vi "PM5000_ReadG6.vi"(6 "DEMO":bool=TRUE, 7 "ID_MEDICION":i32, 8 "error in (no error)":errorcluster, 10 "Equipo_Medicion":T1) -> (0 "error out":errorcluster, 2 "PM_out":T2={"Equipo_Medicion"={"ID_EQUIPO"=0, "IP_EQUIPO"="", "NOMBRE_EQUIPO"="", "ESTADO_EQUIPO"="", "DESCRIPCION"="", "ID_MEDICION"=0, "ESTADO_MEDICION"="", "TIEMPO_MEDICION"="12-02-2019 18:41"}, "VIF_cluster"={"VL_VL"={"V1_V2"=0.0, "V2_V3"=0.0, "V3_V1"=0.0, "Avg_VL_VL"=0.0}, "IL_IL"={"I1"=0.0, "I2"=0.0, "I3"=0.0, "Avg_Amps"=0.0}, "Frecuency"=0.0, "Avg_Frecuency"=0.0}, "Power_cluster"={"Real Power (kW)"={"L1_kW"=0.0, "L2_kW"=0.0, "L3_kW"=0.0, "Total_kW"=0.0}, "Reactive Power (kVAR)"={"L1_kVAR"=0.0, "L2_kVAR"=0.0, "L3_kVAR"=0.0, "Total_kVAR"=0.0}, "Aparent Power (kVA)"={"L1_kVA"=0.0, "L2_kVA"=0.0, "L3_kVA"=0.0, "Total_kVA"=0.0}, "Power Factor (%)"={"L1_PF"=0.0, "L2_PF"=0.0, "L3_PF"=0.0, "Total_PF"=0.0}}, "THD_cluster"={"V_THD"={"V1_V2_THD"=0.0, "V2_V3_THD"=0.0, "V3_V1_THD"=0.0, "Avg_V_V_THD"=0.0}, "I_THD"={"I1_THD"=0.0, "I2_THD"=0.0, "I3_THD"=0.0, "I4_THD"=0.0, "Avg_I_THD"=0.0}}, "Polar_cluster"={"V_polar"={"V1_ang"=0.0, "V1_mag"=0.0, "V2_ang"=0.0, "V2_mag"=0.0, "V3_ang"=0.0, "V3_mag"=0.0}, "I_polar"={"I1_ang"=0.0, "I1_mag"=0.0, "I2_ang"=0.0, "I2_mag"=0.0, "I3_ang"=0.0, "I3_mag"=0.0}}})   [LabVIEW 2018]
uses:
  Controls/Cluster_Data.ctl
  Controls/Equipos_Medicion_cluster.ctl
  Controls/VIF_cluster.ctl
  Controls/Power_cluster.ctl
  Controls/THD_cluster.ctl
  Controls/Polar_cluster.ctl
  Controls/Cluster_HMI_VIFP - 2.ctl
  <vilib>/RAFA Solutions/Harmony UI Controls Kit/Numeric/Horizontal Progress Bar.ctl
  <vilib>/RAFA Solutions/Harmony UI Controls Kit/Numeric/Numeric Indicator.ctl
  Global/globalGenerador6_HMI.vi
  <vilib>/RAFA Solutions/Harmony UI Controls Kit/Flat UI Design.lvlib
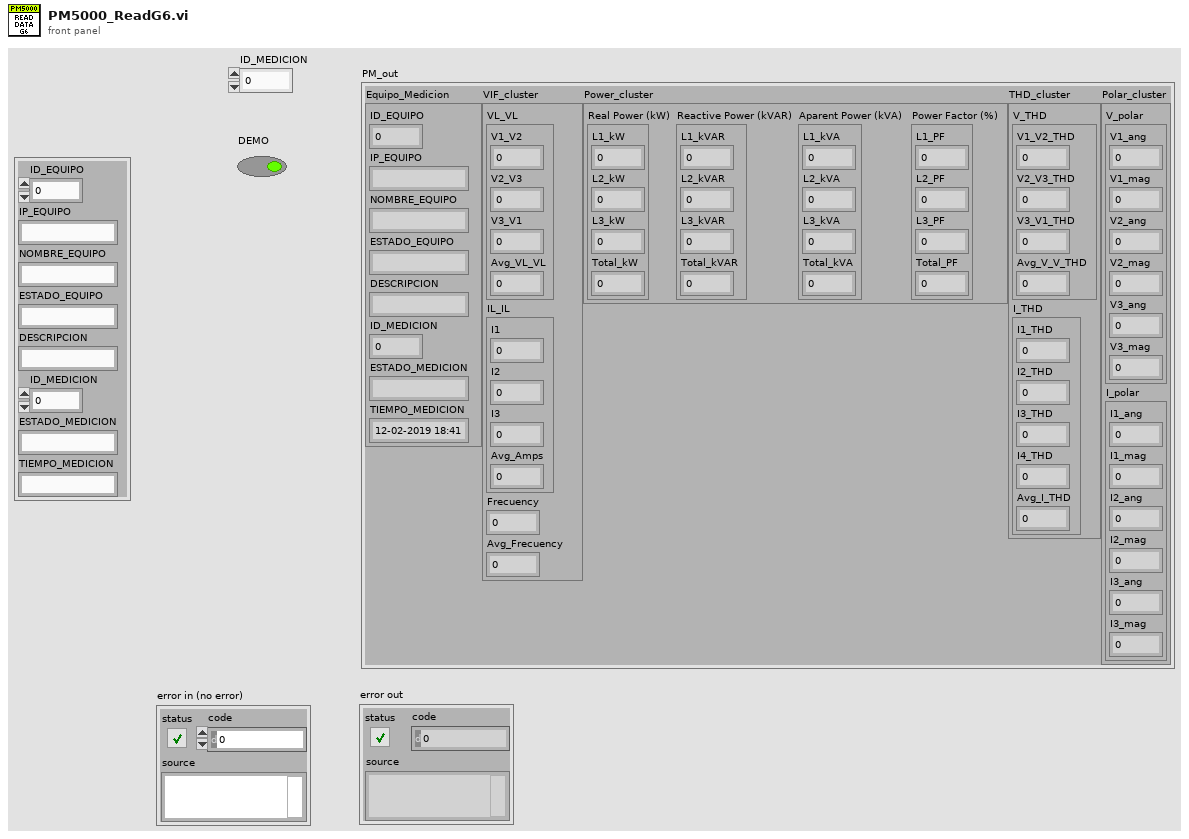
[diagram p1: front panel]
types:
  T1 = typedef "Equipos_Medicion_cluster.ctl" = cluster{"ID_EQUIPO":i32, "IP_EQUIPO":string, "NOMBRE_EQUIPO":string, "ESTADO_EQUIPO":string, "DESCRIPCION":string, "ID_MEDICION":i32, "ESTADO_MEDICION":string, "TIEMPO_MEDICION":string}
  T2 = typedef "Cluster_Data.ctl" = cluster{"Equipo_Medicion":T1, "VIF_cluster":T3, "Power_cluster":T4, "THD_cluster":T5, "Polar_cluster":T6}
  T3 = typedef "VIF_cluster.ctl" = cluster{"VL_VL":cluster{"V1_V2":sgl, "V2_V3":sgl, "V3_V1":sgl, "Avg_VL_VL":sgl}, "IL_IL":cluster{"I1":sgl, "I2":sgl, "I3":sgl, "Avg_Amps":sgl}, "Frecuency":sgl, "Avg_Frecuency":sgl}
  T4 = typedef "Power_cluster.ctl" = cluster{"Real Power (kW)":cluster{"L1_kW":sgl, "L2_kW":sgl, "L3_kW":sgl, "Total_kW":sgl}, "Reactive Power (kVAR)":cluster{"L1_kVAR":sgl, "L2_kVAR":sgl, "L3_kVAR":sgl, "Total_kVAR":sgl}, "Aparent Power (kVA)":cluster{"L1_kVA":sgl, "L2_kVA":sgl, "L3_kVA":sgl, "Total_kVA":sgl}, "Power Factor (%)":cluster{"L1_PF":sgl, "L2_PF":sgl, "L3_PF":sgl, "Total_PF":sgl}}
  T5 = typedef "THD_cluster.ctl" = cluster{"V_THD":cluster{"V1_V2_THD":sgl, "V2_V3_THD":sgl, "V3_V1_THD":sgl, "Avg_V_V_THD":sgl}, "I_THD":cluster{"I1_THD":sgl, "I2_THD":sgl, "I3_THD":sgl, "I4_THD":sgl, "Avg_I_THD":sgl}}
  T6 = typedef "Polar_cluster.ctl" = cluster{"V_polar":cluster{"V1_ang":sgl, "V1_mag":sgl, "V2_ang":sgl, "V2_mag":sgl, "V3_ang":sgl, "V3_mag":sgl}, "I_polar":cluster{"I1_ang":sgl, "I1_mag":sgl, "I2_ang":sgl, "I2_mag":sgl, "I3_ang":sgl, "I3_mag":sgl}}
  T7 = typedef "Cluster_HMI_VIFP - 2.ctl" = cluster{"L2":T8, "L3":T8, "I2":T8, "I3":T8, "Frecuencia [Hz]":T9, "Potencia Total [kW]":T9, "Factor de Potencia":T9, "L1":T8, "I1":T8}
  T8 = typedef "Flat UI Design.lvlib/Horizontal Progress Bar.ctl" = sgl
  T9 = typedef "Flat UI Design.lvlib/Numeric Indicator.ctl" = sgl
  T10 = cluster{"Real Power (kW)":cluster{"L1_kW":sgl, "L2_kW":sgl, "L3_kW":sgl, "Total_kW":sgl}, "Reactive Power (kVAR)":cluster{"L1_kVAR":sgl, "L2_kVAR":sgl, "L3_kVAR":sgl, "Total_kVAR":sgl}, "Aparent Power (kVA)":cluster{"L1_kVA":sgl, "L2_kVA":sgl, "L3_kVA":sgl, "Total_kVA":sgl}, "Power Factor":cluster{"L1_PF":sgl, "L2_PF":sgl, "L3_PF":sgl, "Total_PF":sgl}}
  T11 = cluster{"V_polar":cluster{"V1_ang":sgl, "V1_mag":sgl, "V2_ang":sgl, "V2_mag":sgl, "V3_ang":sgl, "V3_mag":sgl}, "I_polar":cluster{"I1_ang":sgl, "I1_mag":sgl, "I2_ang":sgl, "I2_mag":sgl, "I3_ang":sgl, "I3_mag":sgl}}
  T12 = cluster{"V1_V2":sgl, "V2_V3":sgl, "V3_V1":sgl, "Avg_VL_VL":sgl}
  T13 = cluster{"I1":sgl, "I2":sgl, "I3":sgl, "Avg_Amps":sgl}
  T14 = cluster{"Real Power (kW)":cluster{"L1_kW":sgl, "L2_kW":sgl, "L3_kW":sgl, "Total_kW":sgl}, "Reactive Power (kVAR)":cluster{"L1_kVAR":sgl, "L2_kVAR":sgl, "L3_kVAR":sgl, "Total_kVAR":sgl}, "Aparent Power (kVA)":cluster{"L1_kVA":sgl, "L2_kVA":sgl, "L3_kVA":sgl, "Total_kVA":sgl}, "Power Factor (%)":cluster{"L1_PF":sgl, "L2_PF":sgl, "L3_PF":sgl, "Total_PF":sgl}}
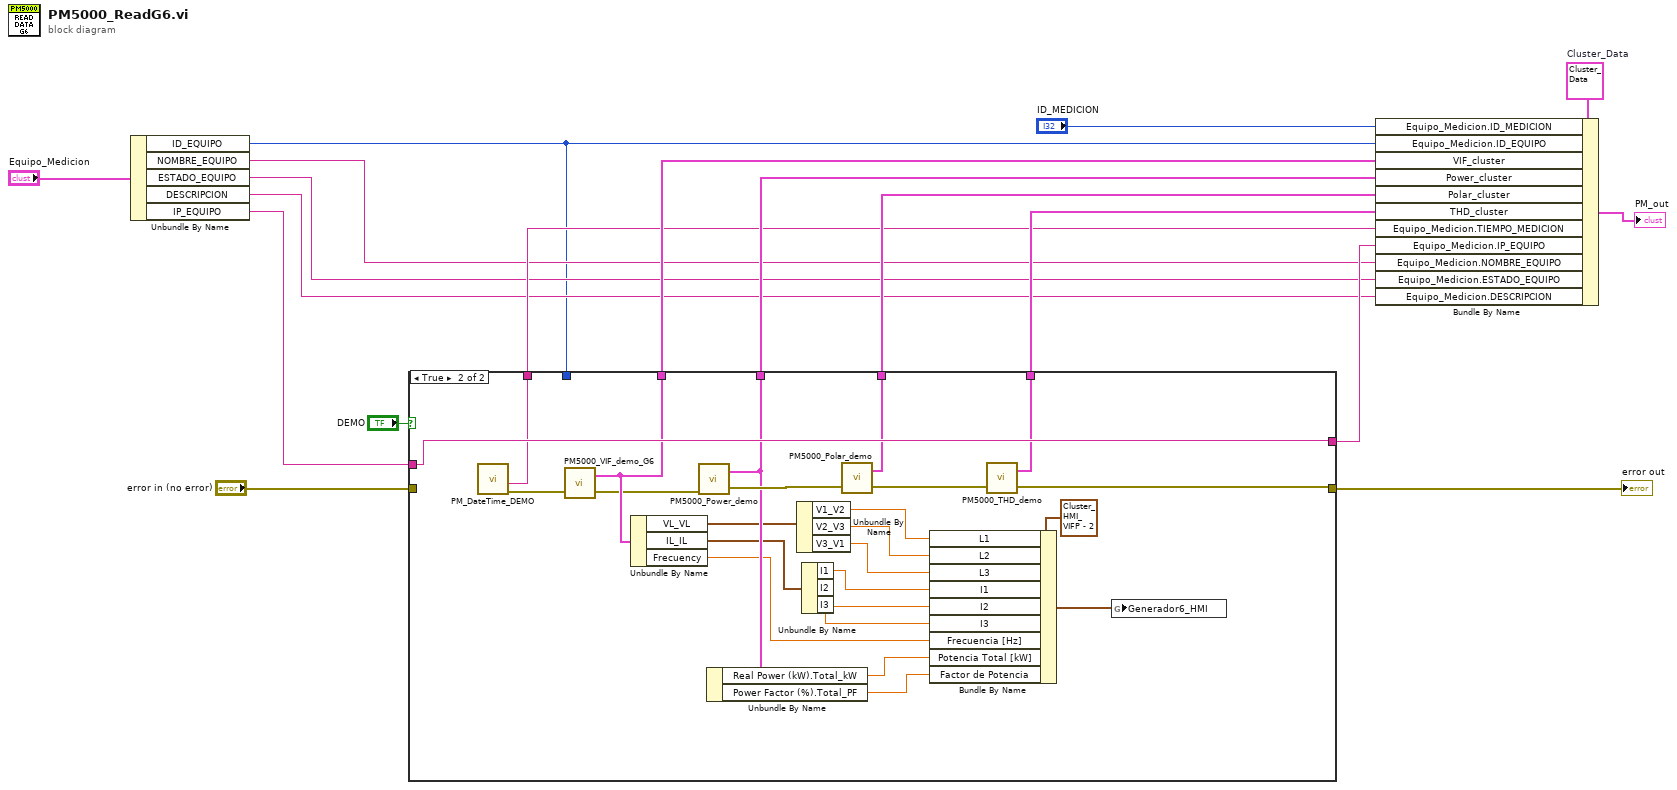
[diagram p0: block diagram]
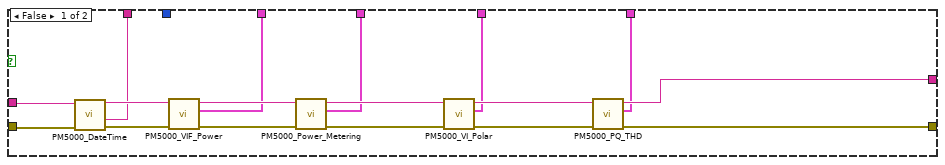
[diagram p2: hidden frame]
diagram:
  w10 = T2 {"Equipo_Medicion"={"ID_EQUIPO"=0, "IP_EQUIPO"="", "NOMBRE_EQUIPO"="", "ESTADO_EQUIPO"="", "DESCRIPCION"="", "ID_MEDICION"=0, "ESTADO_MEDICION"="", "TIEMPO_MEDICION"="12-02-2019 18:41"}, "VIF_cluster"={"VL_VL"={"V1_V2"=0.0, "V2_V3"=0.0, "V3_V1"=0.0, "Avg_VL_VL"=0.0}, "IL_IL"={"I1"=0.0, "I2"=0.0, "I3"=0.0, "Avg_Amps"=0.0}, "Frecuency"=0.0, "Avg_Frecuency"=0.0}, "Power_cluster"={"Real Power (kW)"={"L1_kW"=0.0, "L2_kW"=0.0, "L3_kW"=0.0, "Total_kW"=0.0}, "Reactive Power (kVAR)"={"L1_kVAR"=0.0, "L2_kVAR"=0.0, "L3_kVAR"=0.0, "Total_kVAR"=0.0}, "Aparent Power (kVA)"={"L1_kVA"=0.0, "L2_kVA"=0.0, "L3_kVA"=0.0, "Total_kVA"=0.0}, "Power Factor (%)"={"L1_PF"=0.0, "L2_PF"=0.0, "L3_PF"=0.0, "Total_PF"=0.0}}, "THD_cluster"={"V_THD"={"V1_V2_THD"=0.0, "V2_V3_THD"=0.0, "V3_V1_THD"=0.0, "Avg_V_V_THD"=0.0}, "I_THD"={"I1_THD"=0.0, "I2_THD"=0.0, "I3_THD"=0.0, "I4_THD"=0.0, "Avg_I_THD"=0.0}}, "Polar_cluster"={"V_polar"={"V1_ang"=0.0, "V1_mag"=0.0, "V2_ang"=0.0, "V2_mag"=0.0, "V3_ang"=0.0, "V3_mag"=0.0}, "I_polar"={"I1_ang"=0.0, "I1_mag"=0.0, "I2_ang"=0.0, "I2_mag"=0.0, "I3_ang"=0.0, "I3_mag"=0.0}}}  # Cluster_Data
  n1 = Unbundle By Name("Equipo_Medicion") -> ("ID_EQUIPO"=w1:i32, "NOMBRE_EQUIPO"=w6:string, "ESTADO_EQUIPO"=w4:string, "DESCRIPCION"=w5:string, "IP_EQUIPO"=w3:string)
  n2 = case shown="True" "DEMO" {
    tunnel: w3 -> [w25 w56]
    tunnel: "error in (no error)" -> [w26 _]
    tunnel: [w30 w57] -> w16
    tunnel: [w29 w56] -> w8
    tunnel: [w24 w53] -> w11
    tunnel: [w23 w39] -> w15
    tunnel: [w22 w52] -> w14
    tunnel: [w20 w55] -> w13
    tunnel: [w19 w54] -> w12
    tunnel: w1 -> [_ _]
    frame False {
      n3 = call "PM5000_DateTime.vi"("error in"=w26, "Network Path"=w25) -> ("error out"=w27:errorcluster, "TIEMPO_MEDICION"=w24:string, "Network Path out"=w28:string)  [unwired: 6 in, 1 out]
      n4 = call "PM5000_VIF_Power.vi"("error in"=w27, "Network Path"=w28) -> ("error out"=w34:errorcluster, "VIF_cluster"=w23:T3, "Network Path out"=w35:string)  [unwired: 7 in]
      n5 = call "PM5000_Power_Metering.vi"("error in"=w34, "Network Path"=w35) -> ("error out"=w32:errorcluster, "Power Meter Out"=w22:T10, "Network Path out"=w33:string)  [unwired: 6 in, 1 out]
      n6 = call "PM5000_VI_Polar.vi"("error in"=w32, "Network Path"=w33) -> ("error out"=w31:errorcluster, "VI_polar out"=w20:T11, "Network Path out"=w21:string)  [unwired: 6 in, 1 out]
      n7 = call "PM5000_PQ_THD.vi"("error in"=w31, "Network Path"=w21) -> ("error out"=w30:errorcluster, "THD_cluster"=w19:T5, "Network Path out"=w29:string)  [unwired: 6 in, 1 out]
    }
    frame True {
      n8 = call "PM_DateTime_DEMO.vi"() -> ("error out"=w38:errorcluster, "TIEMPO_MEDICION"=w53:string)  [unwired: 10 in]
      n9 = call "PM5000_VIF_demo_G6.vi"("error in (no error)"=w38) -> ("error out"=w37:errorcluster, "VIF_cluster"=w39:T3)  [unwired: 1 in]
      n10 = Unbundle By Name(w39) -> ("VL_VL"=w50:T12, "IL_IL"=w49:T13, "Frecuency"=w42:sgl)
      n11 = call "PM5000_Power_demo.vi"("error in (no error)"=w37) -> ("error out"=w59:errorcluster, "Power Meter Out"=w52:T14)  [unwired: 1 in]
      n12 = Unbundle By Name(w52) -> ("Real Power (kW).Total_kW"=w41:sgl, "Power Factor (%).Total_PF"=w40:sgl)
      n13 = Unbundle By Name(w50) -> ("V1_V2"=w48:sgl, "V2_V3"=w47:sgl, "V3_V1"=w46:sgl)
      n14 = Unbundle By Name(w49) -> ("I1"=w45:sgl, "I2"=w44:sgl, "I3"=w43:sgl)
      n15 = call "PM5000_Polar_demo.vi"("error in (no error)"=w59) -> ("error out"=w58:errorcluster, "VI_polar out"=w55:T11)  [unwired: 1 in]
      n16 = Bundle By Name(cluster=T7 {"L2"=0.0, "L3"=0.0, "I2"=0.0, "I3"=0.0, "Frecuencia [Hz]"=0.0, "Potencia Total [kW]"=0.0, "Factor de Potencia"=0.0, "L1"=0.0, "I1"=0.0} ("Generador_HMI"), "L1"=w48, "L2"=w47, "L3"=w46, "I1"=w45, "I2"=w44, "I3"=w43, "Frecuencia [Hz]"=w42, "Potencia Total [kW]"=w41, "Factor de Potencia"=w40) -> (w36:T7)
      n17 = call "PM5000_THD_demo.vi"("error in (no error)"=w58) -> ("error out"=w57:errorcluster, "THD_cluster"=w54:T5)  [unwired: 1 in]
      n18 = global write "globalGenerador6_HMI.vi" "Generador6_HMI"(w36) -> ()
    }
  }
  "error out" <- w16
  n19 = Bundle By Name(cluster=w10, "Equipo_Medicion.ID_MEDICION"="ID_MEDICION", "Equipo_Medicion.ID_EQUIPO"=w1, "VIF_cluster"=w15, "Power_cluster"=w14, "Polar_cluster"=w13, "THD_cluster"=w12, "Equipo_Medicion.TIEMPO_MEDICION"=w11, "Equipo_Medicion.IP_EQUIPO"=w8, "Equipo_Medicion.NOMBRE_EQUIPO"=w6, "Equipo_Medicion.ESTADO_EQUIPO"=w4, "Equipo_Medicion.DESCRIPCION"=w5) -> (→"PM_out":T2)
